vi "WriteFGVError.vi"(8 "error in (no error)":errorcluster, 10 "0Cv/1St":i32, 11 "Station Action in":refnum<class "Station Action.lvclass">) -> (0 "error out":errorcluster, 3 "Station Action out":refnum<class "Station Action.lvclass">)   [LabVIEW 2019, in "Station Action.lvclass"]
uses:
  Station Action.lvclass
  Ctrl/Auto Inspection Data Name.ctl
  Ctrl/Auto Inspection Station Name2.ctl
  a048252d-96ea-49cb-9ebf-2aab5575716e.vi
  <vilib>/JDP Science/JSONtext/Variant to JSON Text.vi
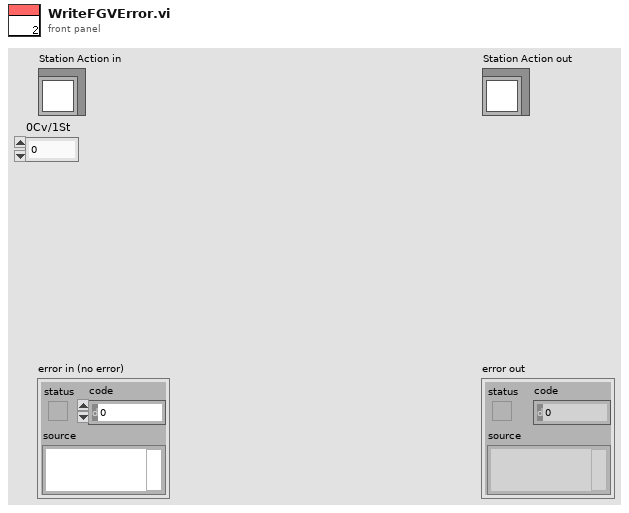
[diagram p1: front panel]
types:
  T1 = typedef "Auto Inspection Data Name.ctl" = enum16{"LocalRun", "ItemSN(TimeCode)", "CurrentAction", "Error", "Data", "OKNG", "電壓值", "電壓值判斷", "電流值", "電流值判斷", "Laser1 Data", "Laser2 Data", "Laser OKNG", "StationNO"}
  T2 = typedef "Auto Inspection Station Name2.ctl" = enum16{"S1Barcode", "S2Measure", "S3Measure", "S4Measure", "S5Measure", "S11_LaserCheck", "S8_Vision AI"}
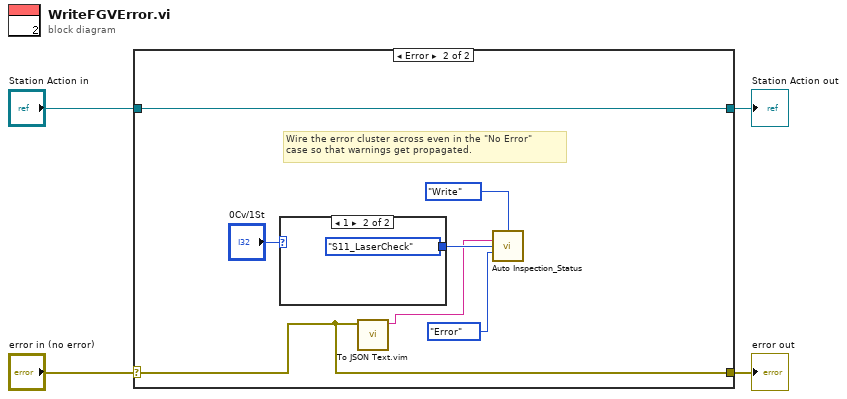
[diagram p0: block diagram]
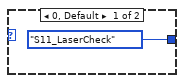
[diagram p3: hidden frame]
diagram:
  n1 = case shown="Error" "error in (no error)" {
    selector: "error in (no error)" -> [w6 w7]
    tunnel: [w6 w7] -> w3
    tunnel: [w5 w13] -> w1
    tunnel: "Station Action in" -> [w5 w13]
    frame No Error {
    }
    frame Error {
      # "Wire the error cluster across even in the \"No Error\"\ncase so that warnings get propagated."
      n2 = case shown="1" "0Cv/1St" {
        tunnel: [Auto_Inspection_Station_Name2."S11_LaserCheck" ("Station") Auto_Inspection_Station_Name2."S11_LaserCheck" ("Station")] -> w11
        frame 0, Default {
        }
        frame 1 {
        }
      }
      n3 = call "To JSON Text.vim"("Anything"=w7) -> ("<JSON>"=w8:string)  [unwired: 9 in, 1 out]
      n4 = call "Auto Inspection_Status.vi"("Action"=enum16{"Initial", "Write", "Read"}."Write", "DataIn"=w8, "Station"=w11, "Data"=Auto_Inspection_Data_Name."Error") -> ()  [unwired: 9 in, 3 out]
    }
  }
  "error out" <- w3
  "Station Action out" <- w1
